vi "Core-DequeueCommands.vi"(8 "error in (no error)":errorcluster, 11 "Engine in":refnum<class "Engine.lvclass">) -> (0 "error out":errorcluster, 2 "Quit?":bool, 3 "Engine out":refnum<class "Engine.lvclass">)   [LabVIEW 2020, in "GLF.lvlib" / "Engine.lvclass"]
uses:
  Engine.lvclass
  Engine.lvclass/Engine.ctl
  Window/Window.lvclass
  Command-CreateWindow--cluster.ctl
  IAmGLF/IAmGLF.lvclass
  IAmGLF/InstanciationNotifierData--cluster.ctl
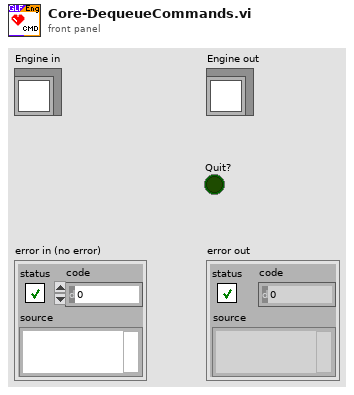
[diagram p1: front panel]
types:
  T1 = typedef "GLF.lvlib/Engine.lvclass/Command-CreateWindow--cluster.ctl" = cluster{"Window Type":refnum<class "Window.lvclass">, "Error Return Notifier":refnum<notifier>}
  T2 = typedef "GLF.lvlib/Engine.lvclass/Command--queue.ctl" = refnum<queue>
  T3 = typedef "GLF.lvlib/Engine.lvclass/Command--cluster.ctl" = cluster{"Cmd":T4, "Data":variant}
  T4 = typedef "GLF.lvlib/Engine.lvclass/Command--enum.ctl" = enum16{"Quit", "Create Window"}
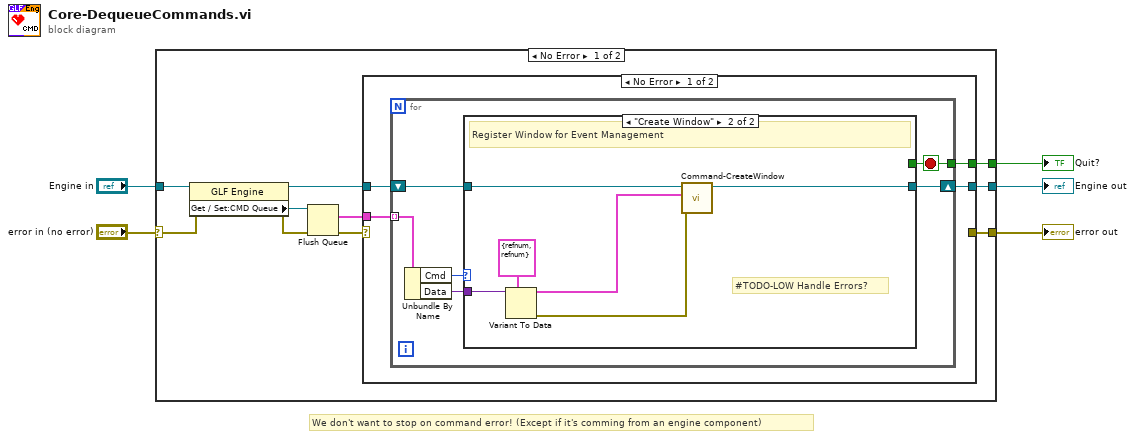
[diagram p0: block diagram]
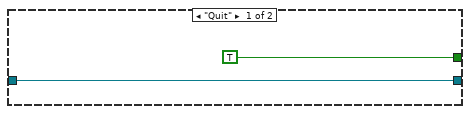
[diagram p2: hidden frame]
diagram:
  # "We don't want to stop on command error! (Except if it's comming from an engine component)"
  n1 = case shown="No Error" "error in (no error)" {
    selector: "error in (no error)" -> [w10 w36]
    tunnel: [w15 w36] -> w2
    tunnel: [w14 _] -> w5
    tunnel: "Engine in" -> [w13 w37]
    tunnel: [w12 w37] -> w3
    frame No Error {
      n2 = property class="GLF Engine"(reference=w13, error in=w10) -> (reference out=w11:refnum<class "Engine.lvclass">, error out=w9:errorcluster, "Get / Set:CMD Queue"=w8:T2)
      n3 = Flush Queue(queue=w8, error in (no error)=w9) -> (remaining elements=w7:T3[], error out=w6:errorcluster)  [unwired: 1 out]
      n4 = case shown="No Error" w6 {
        selector: w6 -> [_ w35]
        tunnel: w7 -> [w19 _]
        tunnel: [_ w35] -> w15
        tunnel: [w18 _] -> w14
        tunnel: w11 -> [w17 w34]
        tunnel: [w16 w34] -> w12
        frame No Error {
          n5 = for {
            tunnel: w19 -> [w25] mode=indexing
            shift-right: [w23] -> w16
            shift-left: w17 -> [w24]
            tunnel: [w21] -> w18
            stop <- w21 stop-if-true
            n6 = Unbundle By Name(w25) -> ("Cmd"=w22:T4, "Data"=w20:variant)
            n7 = case shown="\"Create Window\"" w22 {
              tunnel: w24 -> [w27 w31]
              tunnel: [w27 w29] -> w23
              tunnel: [TRUE _] -> w21
              tunnel: w20 -> [_ w33]
              frame "Quit" {
              }
              frame "Create Window" {
                # "#TODO-LOW Handle Errors?"
                # "Register Window for Event Management"
                n8 = Variant To Data(type=T1 {"Window Type"=refnum, "Error Return Notifier"=refnum} ("Data"), Variant=w33) -> (data=w30:T1, error out=w28:errorcluster)  [unwired: 1 in]
                n9 = call "Command-CreateWindow.vi"("error in (no error)"=w28, "Data"=w30, "Engine in"=w31) -> ("Engine out"=w29:refnum<class "Engine.lvclass">)  [unwired: 8 in]
              }
            }
          }
        }
        frame Error {
        }
      }
    }
    frame Error {
    }
  }
  "error out" <- w2
  "Engine out" <- w3
  "Quit?" <- w5
